vi "Segment players (SubVI).vi"(2 "error In":errorcluster, 3 "Image In":T1) -> (0 "error out":errorcluster, 1 "Image Out":T1)   [LabVIEW 2013]
uses:
  <vilib>/vision/Image Controls.llb/IMAQ Image.ctl
  <vilib>/vision/NI_Vision_Development_Module.lvlib
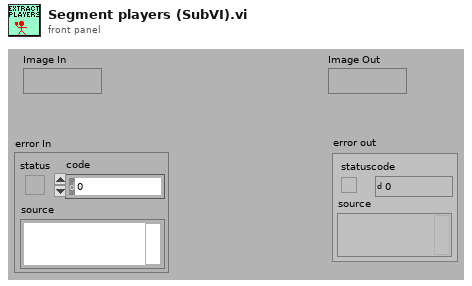
[diagram p1: front panel]
types:
  T1 = typedef "IMAQ Image.ctl" = refnum<image>
  T2 = enum32{"AutoM", "Close", "Dilate", "Erode", "Gradient", "Gradient out", "Gradient in", "Hit miss", "Open", "PClose", "POpen", "Thick", "Thin"}
  T3 = enum32{"AutoM", "Close", "Dilate", "Erode", "Gradient", "Gradient in", "Gradient out", "HitMiss", "Open", "PClose", "POpen", "Thick", "Thin"}
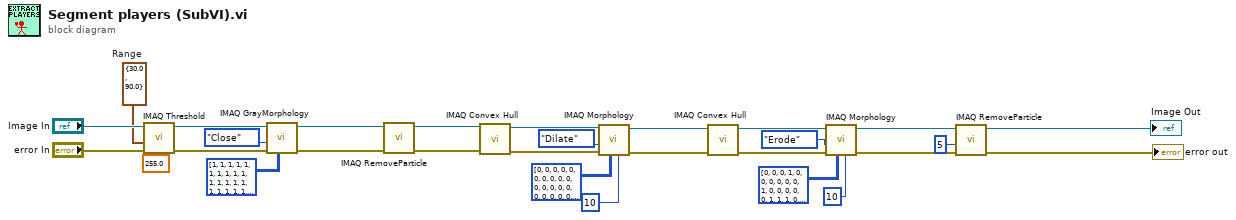
[diagram p0: block diagram]
diagram:
  w7 = cluster{"Lower value":sgl, "Upper value":sgl} {"Lower value"=30.0, "Upper value"=90.0}  # Range
  n1 = call "IMAQ Threshold"("Replace Value"=sgl 255.0, "error in (no error)"="error In", "Range"=w7, "Image Src"="Image In") -> ("error out"=w12:errorcluster, "Image Dst Out"=w8:T1)  [unwired: 6 in]
  n2 = call "IMAQ GrayMorphology"("Structuring Element"=i32[][] [[1, 1, 1, 1, 1, 1, 1, 1, 1], [1, 1, 1, 1, 1, 1, 1, 1, 1], [1, 1, 1, 1, 1, 1, 1, 1, 1], [1, 1, 1, 1, 1, 1, 1, 1, 1], [1, 1, 1, 1, 1, 1, 1, 1, 1], [1, 1, 1, 1, 1, 1, 1, 1, 1], [1, 1, 1, 1, 1, 1, 1, 1, 1], [1, 1, 1, 1, 1, 1, 1, 1, 1], [1, 1, 1, 1, 1, 1, 1, 1, 1]], "error in (no error)"=w12, "Operation"=T3."Close", "Image Src"=w8) -> ("error out"=w14:errorcluster, "Image Dst Out"=w13:T1)  [unwired: 6 in]
  n3 = call "IMAQ RemoveParticle"("error in (no error)"=w14, "Image Src"=w13) -> ("error out"=w15:errorcluster, "Image Dst Out"=w16:T1)  [unwired: 8 in]
  n4 = call "IMAQ Convex Hull"("error in (no error)"=w15, "Image Src"=w16) -> ("error out"=w19:errorcluster, "Image Dst Out"=w29:T1)  [unwired: 8 in]
  n5 = call "IMAQ Morphology"("Number of iterations (1)"=10, "Structuring Element"=i32[][] [[0, 0, 0, 0, 0, 0, 0], [0, 0, 0, 0, 0, 0, 0], [0, 0, 0, 0, 0, 0, 0], [0, 0, 0, 0, 0, 0, 0], [0, 0, 1, 1, 1, 0, 0], [0, 0, 0, 1, 0, 0, 0], [0, 0, 0, 1, 0, 0, 0]], "error in (no error)"=w19, "Operation"=T2."Dilate", "Image Src"=w29) -> ("error out"=w25:errorcluster, "Image Dst Out"=w24:T1)  [unwired: 5 in]
  n6 = call "IMAQ Convex Hull"("error in (no error)"=w25, "Image Src"=w24) -> ("error out"=w27:errorcluster, "Image Dst Out"=w26:T1)  [unwired: 8 in]
  n7 = call "IMAQ Morphology"("Number of iterations (1)"=10, "Structuring Element"=i32[][] [[0, 0, 0, 1, 0, 0, 0], [0, 0, 0, 1, 0, 0, 0], [0, 0, 1, 1, 1, 0, 0], [0, 0, 0, 0, 0, 0, 0], [0, 0, 0, 0, 0, 0, 0], [0, 0, 0, 0, 0, 0, 0], [0, 0, 0, 0, 0, 0, 0]], "error in (no error)"=w27, "Operation"=T2."Erode", "Image Src"=w26) -> ("error out"=w4:errorcluster, "Image Dst Out"=w5:T1)  [unwired: 5 in]
  n8 = call "IMAQ RemoveParticle"("error in (no error)"=w4, "Number of Erosion"=5, "Image Src"=w5) -> ("error out"=→"error out":errorcluster, "Image Dst Out"=→"Image Out":T1)  [unwired: 7 in]
